vi "Test - Normalise Vector.vi"() -> ()   [LabVIEW 2020, in "3D (FPGA).lvlib"]
uses:
  3D (FPGA).lvlib
  Vector 3D.ctl
panel:
  out "Vector 3D Normalised":T1
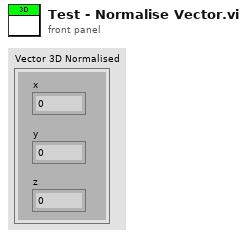
[diagram p1: front panel]
types:
  T1 = typedef "3D (FPGA).lvlib/Vector 3D.ctl" = cluster{"x":sgl, "y":sgl, "z":sgl}
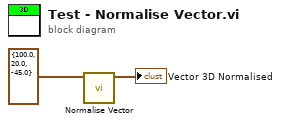
[diagram p0: block diagram]
diagram:
  n1 = call "Normalise Vector.vi"("Vector 3D"=T1 {"x"=100.0, "y"=20.0, "z"=-45.0}) -> ("Vector 3D Normalised"=→"Vector 3D Normalised":T1)  [unwired: 10 in]
